vi "upload.sign_and_start_upload.vi"(8 "error in":errorcluster, 10 "Multipart Upload in":refnum<class "Multipart Upload.lvclass">) -> (0 "error out":errorcluster, 2 "Multipart Upload out":refnum<class "Multipart Upload.lvclass">)   [LabVIEW 2020]
uses:
  Nominal Client.lvclass/Nominal Client.ctl
  Nominal Client MultiPart Upload/Multipart Upload.lvclass/Multipart Upload.ctl
  Nominal Client MultiPart Upload/Multipart Upload.lvclass
panel:
  in  "File Part Binary":string
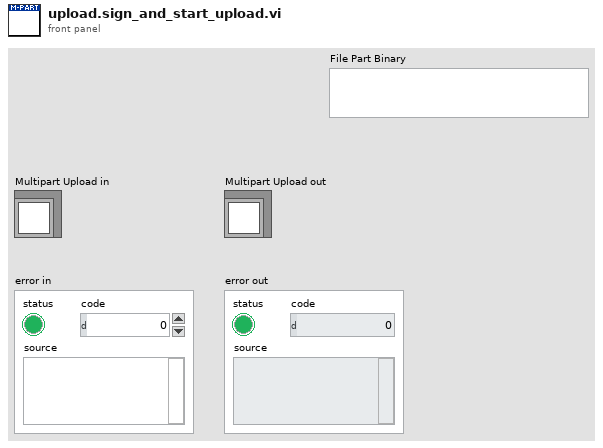
[diagram p1: front panel]
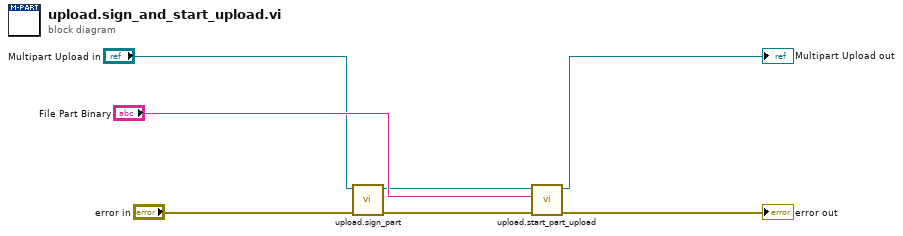
[diagram p0: block diagram]
diagram:
  n1 = call "upload.sign_part.vi"("error in"="error in", "Multipart Upload in"="Multipart Upload in") -> ("error out"=w7:errorcluster, "Multipart Upload out"=w3:refnum<class "Multipart Upload.lvclass">)  [unwired: 8 in]
  n2 = call "upload.start_part_upload.vi"("error in"=w7, "File Part Binary"="File Part Binary", "Multipart Upload"=w3) -> ("error out"=→"error out":errorcluster, "Multipart Upload out"=→"Multipart Upload out":refnum<class "Multipart Upload.lvclass">)  [unwired: 7 in]
